vi "Protocol Init.vi"(4 "error in (no error)":errorcluster, 7 "connection ID":refnum<k5>) -> (0 "Message length":i32, 1 "error out":errorcluster, 2 "connection ID out":refnum<k5>, 3 "Number of messages":i32)   [LabVIEW 2017]
panel:
  # "This SubVI will get the initial\nparameters of the command\nsent by Cockpit\n- message length (message of length 4)\n- number of messages of that length"
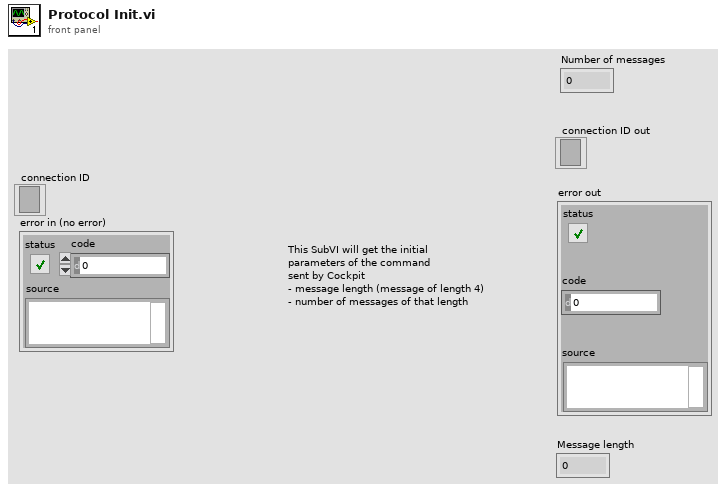
[diagram p1: front panel]
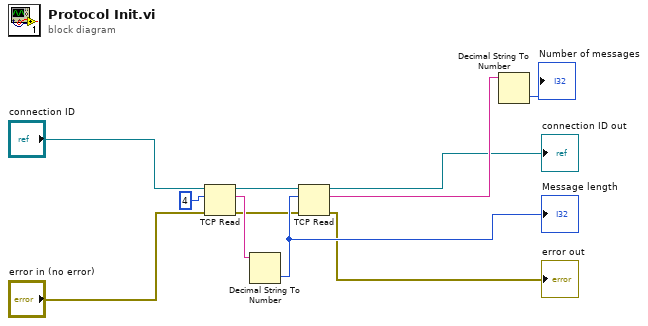
[diagram p0: block diagram]
diagram:
  n1 = TCP Read(connection ID="connection ID", bytes to read=4, error in (no error)="error in (no error)") -> (connection ID out=w11:refnum<k5>, data out=w9:string, error out=w4:errorcluster)  [unwired: 2 in]
  n2 = Decimal String To Number(string=w9) -> (number=w7:i32)  [unwired: 2 in, 1 out]
  "Message length" <- w7
  n3 = TCP Read(connection ID=w11, bytes to read=w7, error in (no error)=w4) -> (connection ID out=→"connection ID out":refnum<k5>, data out=w8:string, error out=→"error out":errorcluster)  [unwired: 2 in]
  n4 = Decimal String To Number(string=w8) -> (number=→"Number of messages":i32)  [unwired: 2 in, 1 out]
